vi "Example Graph.vi"() -> ()   [LabVIEW 2010]
uses:
  C:/tf/play/labview/Tinkerforge.dll
panel:
  in  "stop":bool
  out "graph":sgl[](graph)
  in  "uid":string="amb"
  in  "port":i32=4223
  in  "host":string="localhost"
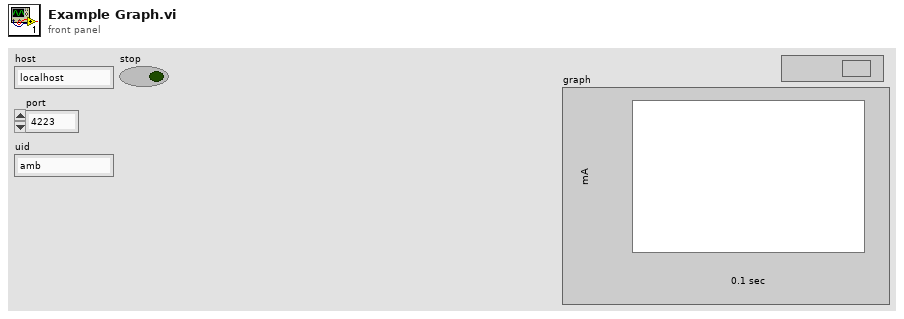
[diagram p1: front panel]
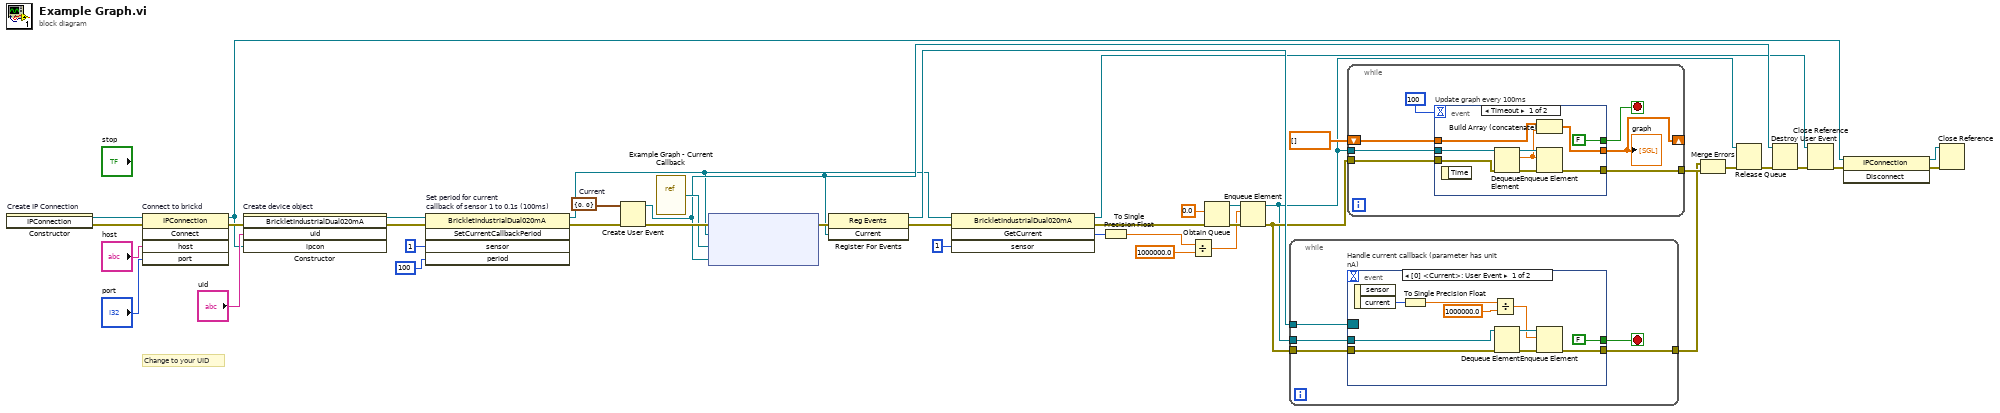
[diagram p0: block diagram]
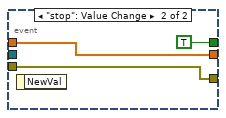
[diagram p2: hidden frame]
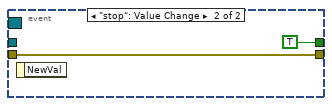
[diagram p3: hidden frame]
diagram:
  w26 = cluster{"sensor":u8, "current":i32} {"sensor"=0, "current"=0}  # Current
  # "Change to your UID"
  n1 = constructor on="Create IP Connection" class="IPConnection"() -> (reference out=w41:refnum<k24>, error out=w11:errorcluster)  [unwired: 3 in, 1 out]
  n2 = invoke on="Connect to brickd" class="IPConnection" method="Connect"(reference=w41, error in=w11, "host"="host", "port"="port") -> (reference out=w34:refnum<k24>, error out=w37:errorcluster)  [unwired: 1 in, 3 out]
  n3 = constructor on="Create device object" class="BrickletIndustrialDual020mA"(error in=w37, "uid"="uid", "ipcon"=w34) -> (reference out=w23:refnum<k24>, error out=w25:errorcluster)  [unwired: 2 in, 3 out]
  n4 = invoke on="Set period for current\ncallback of sensor 1 to 0.1s (100ms)" class="BrickletIndustrialDual020mA" method="SetCurrentCallbackPeriod"(reference=w23, error in=w25, "sensor"=u8 1, "period"=i64 100) -> (reference out=w8:refnum<k24>, error out=w24:errorcluster)  [unwired: 1 in, 3 out]
  n5 = Create User Event(user event datatype=w26, error in=w24) -> (user event=w28:refnum<user-event>, error out=w32:errorcluster)
  n6 = vi-ref "Example Graph - Current Callback.vi"() -> ("vi reference"=w30:refnum<vi>)
  n7 = node ("Register Event Callback")(w32, w8, w30, w28) -> (w31:errorcluster)  [unwired: 1 in, 1 out]
  n8 = register-events(error in=w31, w28) -> (reference out=w29:refnum<event-registration>, error out=w10:errorcluster)  [unwired: 1 in]
  n9 = invoke class="BrickletIndustrialDual020mA" method="GetCurrent"(reference=w8, error in=w10, "sensor"=u8 1) -> (reference out=w7:refnum<k24>, error out=w9:errorcluster, "GetCurrent"=w4:i32)  [unwired: 1 in, 1 out]
  n10 = To Single Precision Float(number=w4) -> (single precision float=w6:sgl)
  n11 = Divide(x=w6, y=sgl 1000000.0) -> (x/y=w3:sgl)
  n12 = Obtain Queue(element data type=sgl 0.0, error in (no error)=w9) -> (queue out=w15:refnum<queue>, error out=w17:errorcluster)  [unwired: 3 in, 1 out]
  n13 = Enqueue Element(queue=w15, element=w3, error in (no error)=w17) -> (queue out=w12:refnum<queue>, error out=w16:errorcluster)  [unwired: 1 in, 1 out]
  n14 = while {
    tunnel: w29 -> [w46]
    tunnel: [w44] -> w20
    tunnel: w16 -> [w45]
    tunnel: w12 -> [w43]
    stop <- w42 stop-if-true
    n15 = event "Handle current callback (parameter has unit nA)" shown="[0] <Current>: User Event" {
      selector: w46 -> [_ _]
      dyn-events: _ -> [_ _]
      timeout: _ -> [_ _]
      tunnel: w45 -> [w54 w57]
      tunnel: [w52 w57] -> w44
      tunnel: w43 -> [w51 _]
      tunnel: [FALSE TRUE] -> w42
      event User Event {
        n16 = event-data() -> ("current"=w47:i32)  [unwired: 1 in, 1 out]
        n17 = To Single Precision Float(number=w47) -> (single precision float=w55:sgl)
        n18 = Divide(x=w55, y=sgl 1000000.0) -> (x/y=w49:sgl)
        n19 = Dequeue Element(queue=w51, error in (no error)=w54) -> (queue out=w50:refnum<queue>, error out=w53:errorcluster)  [unwired: 1 in, 2 out]
        n20 = Enqueue Element(queue=w50, element=w49, error in (no error)=w53) -> (error out=w52:errorcluster)  [unwired: 1 in, 2 out]
      }
      event "stop": Value Change {
        n21 = event-data() -> ()  [unwired: 1 in, 1 out]
      }
    }
  }
  n22 = while {
    tunnel: [w61] -> w21
    tunnel: w16 -> [w62]
    shift-right: [w63] -> _
    shift-left: sgl[] [] -> [w64]
    tunnel: w12 -> [w60]
    stop <- w59 stop-if-true
    n23 = event "Update graph every 100ms" shown="[0] Timeout" {
      selector: _ -> [_ _]
      dyn-events: _ -> [_ _]
      timeout: 100 -> [_ _]
      tunnel: [w74 w76] -> w63
      tunnel: w64 -> [w67 w76]
      tunnel: w62 -> [w73 w75]
      tunnel: [w70 w75] -> w61
      tunnel: w60 -> [w72 _]
      tunnel: [FALSE TRUE] -> w59
      event Timeout {
        n24 = event-data() -> ()  [unwired: 1 in, 1 out]
        n25 = Dequeue Element(queue=w72, error in (no error)=w73) -> (queue out=w69:refnum<queue>, element=w68:sgl, error out=w71:errorcluster)  [unwired: 1 in, 1 out]
        n26 = Build Array (concatenate)(w67, w68) -> (w74:sgl[])
        n27 = Enqueue Element(queue=w69, element=w68, error in (no error)=w71) -> (error out=w70:errorcluster)  [unwired: 1 in, 2 out]
      }
      event "stop": Value Change {
        n28 = event-data() -> ()  [unwired: 1 in, 1 out]
      }
    }
    "graph" <- w63
  }
  n29 = Merge Errors(w20, w21) -> (w14:errorcluster)
  n30 = Release Queue(queue=w12, error in (no error)=w14) -> (error out=w13:errorcluster)  [unwired: 1 in, 2 out]
  n31 = Destroy User Event(user event=w28, error in=w13) -> (error out=w27:errorcluster)
  n32 = Close Reference(reference=w7, error in (no error)=w27) -> (error out=w36:errorcluster)
  n33 = invoke class="IPConnection" method="Disconnect"(reference=w34, error in=w36) -> (reference out=w33:refnum<k24>, error out=w35:errorcluster)  [unwired: 1 in, 1 out]
  n34 = Close Reference(reference=w33, error in (no error)=w35) -> ()  [unwired: 1 out]
